vi "Ball delete.vi"(4 "error in":errorcluster, 5 "ball hp":i16, 7 "Ball Ref":refnum<vi>) -> (0 "error out":errorcluster, 1 "hp new":i16)   [LabVIEW 2014]
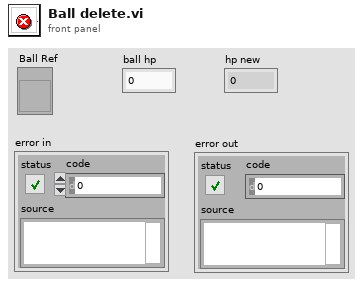
[diagram p1: front panel]
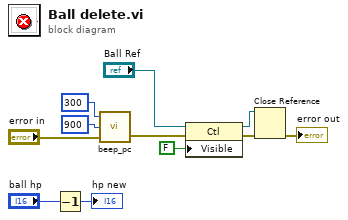
[diagram p0: block diagram]
diagram:
  n1 = Decrement(x="ball hp") -> (x-1=→"hp new":i16)
  n2 = call "beep_pc.vi"("error in"="error in", "Duration (seconds)"=900, "Frequency (Hz)"=300) -> ("error out"=w3:errorcluster)  [unwired: 1 in]
  n3 = property class="Ctl"(reference="Ball Ref", error in=w3, "Visible"=FALSE) -> (reference out=w7:refnum<vi>, error out=w6:errorcluster)
  n4 = Close Reference(reference=w7, error in (no error)=w6) -> (error out=→"error out":errorcluster)
